vi "Wago 4 Station Door Status.vi"(7 "Station 1-4":bool, 8 "error in (no error)":errorcluster, 10 "Wago Data Input":T2 {"Input Process Image"."Software Constants"."Room PID Settings"."Room Dehumid Temperature I (*RM Dehum I1)" max=30000 step=1; "Input Process Image"."Software Constants"."Room PID Settings"."Room Dehumid Temperature P (*RM Dehum P1)" max=30000 step=1; "Input Process Image"."Software Constants"."Room PID Settings"."Room Cool Temperature I (*RM Cool I1)" max=30000 step=1; "Input Process Image"."Software Constants"."Room PID Settings"."Room Cool Temperature P (*RM Cool P1)" max=30000 step=1; "Input Process Image"."Software Constants"."Room PID Settings"."Room Heat I (*RM Heat I1)" max=30000 step=1; "Input Process Image"."Software Constants"."Room PID Settings"."Room Heat P (*RM Heat P1)" max=30000 step=1; "Input Process Image"."Software Constants"."Room PID Settings"."Room Humidity I (*RM Hum I1)" max=30000 step=1; "Input Process Image"."Software Constants"."Room PID Settings"."Room Humidity P (*RM Hum P1)" max=30000 step=1; "Input Process Image"."Software Constants"."Room PID Settings"."Room Dry I (*RM Dry I1)" max=30000 step=1; "Input Process Image"."Software Constants"."Room PID Settings"."Room Dry P(*RM Dry P1)" max=30000 step=1}, 11 "Modbus Master in":refnum<class "Modbus Master.lvclass">) -> (0 "error out":errorcluster, 2 "Wago Data Output":T2 {"Input Process Image"."Software Constants"."Room PID Settings"."Room Dehumid Temperature I (*RM Dehum I1)" max=30000 step=1; "Input Process Image"."Software Constants"."Room PID Settings"."Room Dehumid Temperature P (*RM Dehum P1)" max=30000 step=1; "Input Process Image"."Software Constants"."Room PID Settings"."Room Cool Temperature I (*RM Cool I1)" max=30000 step=1; "Input Process Image"."Software Constants"."Room PID Settings"."Room Cool Temperature P (*RM Cool P1)" max=30000 step=1; "Input Process Image"."Software Constants"."Room PID Settings"."Room Heat I (*RM Heat I1)" max=30000 step=1; "Input Process Image"."Software Constants"."Room PID Settings"."Room Heat P (*RM Heat P1)" max=30000 step=1; "Input Process Image"."Software Constants"."Room PID Settings"."Room Humidity I (*RM Hum I1)" max=30000 step=1; "Input Process Image"."Software Constants"."Room PID Settings"."Room Humidity P (*RM Hum P1)" max=30000 step=1; "Input Process Image"."Software Constants"."Room PID Settings"."Room Dry I (*RM Dry I1)" max=30000 step=1; "Input Process Image"."Software Constants"."Room PID Settings"."Room Dry P(*RM Dry P1)" max=30000 step=1}, 3 "Modbus master out":refnum<class "Modbus Master.lvclass">)   [LabVIEW 2016]
uses:
  <vilib>/NI/Modbus Library/API/Master/Modbus Master.lvclass
  Type Definitions/Wago Main Control.ctl
  Type Definitions/Wago Output Data Process Image.ctl
  Type Definitions/Wago Room Condtions.ctl
  Type Definitions/Wago Door Relays.ctl
  Type Definitions/Wago Contactor Settings.ctl
  Type Definitions/Wago Ground Leakage.ctl
  Type Definitions/Wago Input Process Image.ctl
  Type Definitions/Wago Room PID Settings.ctl
  Type Definitions/Wago Measured Input Data.ctl
  Type Definitions/Wago Room Setpoint Targets.ctl
  Type Definitions/Wago Output Commands.ctl
panel:
  in  "Wago Output Words 24":T1=839 items=["twHeatCtrl"=512, "twSteamCtrl"=513, "twCoolCtrl"=514, "twDehumCtrl"=515, "Output QX4 Bool"=516, "Output QX5 Bool"=517, "Output QX6 Bool"=518, "Output QX7 Bool"=519, "Output QX8 Bool"=520, "Output QX9 Bool"=521, "Output QX10"=522, "twRoomTemp"=840, "twRoomHum"=841, "twSuppTemp"=842, "twCoolTemp"=843, "twDehumTemp"=844, "twGlycolTemp"=845, "twHeatRate"=846, "twSteamRate"=847, "twCoolRate"=848, "twDehumRate"=849, "twStatus"=850, "twDoorEna"=851, "Rm1St1Dr1Stat"=816, "Rm1St2Dr1Stat"=817, "Rm1St3Dr1Stat"=818, "Rm1St4Dr1Stat"=819, "Rm1St5Dr1Stat"=820, "Rm1St6Dr1Stat"=821, "Rm1St7Dr1Stat"=822, "Rm1St8Dr1Stat"=823, "Rm1St1Dr2Stat"=824, "Rm1St2Dr2Stat"=825, "Rm1St3Dr2Stat"=826, "Rm1St4Dr2Stat"=827, "Rm1St5Dr2Stat"=828, "Rm1St6DrStat"=829, "Rm1St7Dr2Stat"=830, "Rm1St8Dr2Stat"=831, "Rm1St1Dr3Stat"=832, "Rm1St2Dr3Stat"=833, "Rm1St3Dr3Stat"=834, "Rm1St4Dr3Stat"=835, "Rm1St5Dr3Stat"=836, "Rm1St6Dr3Stat"=837, "Rm1St7Dr3Stat"=838, "Rm1St8Dr3Stat"=839, "twVoltMon1"=784, "twVoltMon2"=785, "twVoltMon3"=786, "twVoltMon4"=787, "twVoltMon5"=788, "twVoltMon6"=789, "twVoltMon7"=790, "twVoltMon8"=791, "twVoltStat1"=792, "twVoltStat2"=793, "twVoltStat3"=794, "twVoltStat4"=795, "twVoltStat5"=796, "twVoltStat6"=797, "twVoltStat7"=798, "twVoltStat8"=799]
  in  "Wago Output Words 23":T1=831 items=["twHeatCtrl"=512, "twSteamCtrl"=513, "twCoolCtrl"=514, "twDehumCtrl"=515, "Output QX4 Bool"=516, "Output QX5 Bool"=517, "Output QX6 Bool"=518, "Output QX7 Bool"=519, "Output QX8 Bool"=520, "Output QX9 Bool"=521, "Output QX10"=522, "twRoomTemp"=840, "twRoomHum"=841, "twSuppTemp"=842, "twCoolTemp"=843, "twDehumTemp"=844, "twGlycolTemp"=845, "twHeatRate"=846, "twSteamRate"=847, "twCoolRate"=848, "twDehumRate"=849, "twStatus"=850, "twDoorEna"=851, "Rm1St1Dr1Stat"=816, "Rm1St2Dr1Stat"=817, "Rm1St3Dr1Stat"=818, "Rm1St4Dr1Stat"=819, "Rm1St5Dr1Stat"=820, "Rm1St6Dr1Stat"=821, "Rm1St7Dr1Stat"=822, "Rm1St8Dr1Stat"=823, "Rm1St1Dr2Stat"=824, "Rm1St2Dr2Stat"=825, "Rm1St3Dr2Stat"=826, "Rm1St4Dr2Stat"=827, "Rm1St5Dr2Stat"=828, "Rm1St6DrStat"=829, "Rm1St7Dr2Stat"=830, "Rm1St8Dr2Stat"=831, "Rm1St1Dr3Stat"=832, "Rm1St2Dr3Stat"=833, "Rm1St3Dr3Stat"=834, "Rm1St4Dr3Stat"=835, "Rm1St5Dr3Stat"=836, "Rm1St6Dr3Stat"=837, "Rm1St7Dr3Stat"=838, "Rm1St8Dr3Stat"=839, "twVoltMon1"=784, "twVoltMon2"=785, "twVoltMon3"=786, "twVoltMon4"=787, "twVoltMon5"=788, "twVoltMon6"=789, "twVoltMon7"=790, "twVoltMon8"=791, "twVoltStat1"=792, "twVoltStat2"=793, "twVoltStat3"=794, "twVoltStat4"=795, "twVoltStat5"=796, "twVoltStat6"=797, "twVoltStat7"=798, "twVoltStat8"=799]
  in  "Wago Output Words 22":T1=823 items=["twHeatCtrl"=512, "twSteamCtrl"=513, "twCoolCtrl"=514, "twDehumCtrl"=515, "Output QX4 Bool"=516, "Output QX5 Bool"=517, "Output QX6 Bool"=518, "Output QX7 Bool"=519, "Output QX8 Bool"=520, "Output QX9 Bool"=521, "Output QX10"=522, "twRoomTemp"=840, "twRoomHum"=841, "twSuppTemp"=842, "twCoolTemp"=843, "twDehumTemp"=844, "twGlycolTemp"=845, "twHeatRate"=846, "twSteamRate"=847, "twCoolRate"=848, "twDehumRate"=849, "twStatus"=850, "twDoorEna"=851, "Rm1St1Dr1Stat"=816, "Rm1St2Dr1Stat"=817, "Rm1St3Dr1Stat"=818, "Rm1St4Dr1Stat"=819, "Rm1St5Dr1Stat"=820, "Rm1St6Dr1Stat"=821, "Rm1St7Dr1Stat"=822, "Rm1St8Dr1Stat"=823, "Rm1St1Dr2Stat"=824, "Rm1St2Dr2Stat"=825, "Rm1St3Dr2Stat"=826, "Rm1St4Dr2Stat"=827, "Rm1St5Dr2Stat"=828, "Rm1St6DrStat"=829, "Rm1St7Dr2Stat"=830, "Rm1St8Dr2Stat"=831, "Rm1St1Dr3Stat"=832, "Rm1St2Dr3Stat"=833, "Rm1St3Dr3Stat"=834, "Rm1St4Dr3Stat"=835, "Rm1St5Dr3Stat"=836, "Rm1St6Dr3Stat"=837, "Rm1St7Dr3Stat"=838, "Rm1St8Dr3Stat"=839, "twVoltMon1"=784, "twVoltMon2"=785, "twVoltMon3"=786, "twVoltMon4"=787, "twVoltMon5"=788, "twVoltMon6"=789, "twVoltMon7"=790, "twVoltMon8"=791, "twVoltStat1"=792, "twVoltStat2"=793, "twVoltStat3"=794, "twVoltStat4"=795, "twVoltStat5"=796, "twVoltStat6"=797, "twVoltStat7"=798, "twVoltStat8"=799]
  in  "Wago Output Words 21":T1=838 items=["twHeatCtrl"=512, "twSteamCtrl"=513, "twCoolCtrl"=514, "twDehumCtrl"=515, "Output QX4 Bool"=516, "Output QX5 Bool"=517, "Output QX6 Bool"=518, "Output QX7 Bool"=519, "Output QX8 Bool"=520, "Output QX9 Bool"=521, "Output QX10"=522, "twRoomTemp"=840, "twRoomHum"=841, "twSuppTemp"=842, "twCoolTemp"=843, "twDehumTemp"=844, "twGlycolTemp"=845, "twHeatRate"=846, "twSteamRate"=847, "twCoolRate"=848, "twDehumRate"=849, "twStatus"=850, "twDoorEna"=851, "Rm1St1Dr1Stat"=816, "Rm1St2Dr1Stat"=817, "Rm1St3Dr1Stat"=818, "Rm1St4Dr1Stat"=819, "Rm1St5Dr1Stat"=820, "Rm1St6Dr1Stat"=821, "Rm1St7Dr1Stat"=822, "Rm1St8Dr1Stat"=823, "Rm1St1Dr2Stat"=824, "Rm1St2Dr2Stat"=825, "Rm1St3Dr2Stat"=826, "Rm1St4Dr2Stat"=827, "Rm1St5Dr2Stat"=828, "Rm1St6DrStat"=829, "Rm1St7Dr2Stat"=830, "Rm1St8Dr2Stat"=831, "Rm1St1Dr3Stat"=832, "Rm1St2Dr3Stat"=833, "Rm1St3Dr3Stat"=834, "Rm1St4Dr3Stat"=835, "Rm1St5Dr3Stat"=836, "Rm1St6Dr3Stat"=837, "Rm1St7Dr3Stat"=838, "Rm1St8Dr3Stat"=839, "twVoltMon1"=784, "twVoltMon2"=785, "twVoltMon3"=786, "twVoltMon4"=787, "twVoltMon5"=788, "twVoltMon6"=789, "twVoltMon7"=790, "twVoltMon8"=791, "twVoltStat1"=792, "twVoltStat2"=793, "twVoltStat3"=794, "twVoltStat4"=795, "twVoltStat5"=796, "twVoltStat6"=797, "twVoltStat7"=798, "twVoltStat8"=799]
  in  "Wago Output Words 20":T1=830 items=["twHeatCtrl"=512, "twSteamCtrl"=513, "twCoolCtrl"=514, "twDehumCtrl"=515, "Output QX4 Bool"=516, "Output QX5 Bool"=517, "Output QX6 Bool"=518, "Output QX7 Bool"=519, "Output QX8 Bool"=520, "Output QX9 Bool"=521, "Output QX10"=522, "twRoomTemp"=840, "twRoomHum"=841, "twSuppTemp"=842, "twCoolTemp"=843, "twDehumTemp"=844, "twGlycolTemp"=845, "twHeatRate"=846, "twSteamRate"=847, "twCoolRate"=848, "twDehumRate"=849, "twStatus"=850, "twDoorEna"=851, "Rm1St1Dr1Stat"=816, "Rm1St2Dr1Stat"=817, "Rm1St3Dr1Stat"=818, "Rm1St4Dr1Stat"=819, "Rm1St5Dr1Stat"=820, "Rm1St6Dr1Stat"=821, "Rm1St7Dr1Stat"=822, "Rm1St8Dr1Stat"=823, "Rm1St1Dr2Stat"=824, "Rm1St2Dr2Stat"=825, "Rm1St3Dr2Stat"=826, "Rm1St4Dr2Stat"=827, "Rm1St5Dr2Stat"=828, "Rm1St6DrStat"=829, "Rm1St7Dr2Stat"=830, "Rm1St8Dr2Stat"=831, "Rm1St1Dr3Stat"=832, "Rm1St2Dr3Stat"=833, "Rm1St3Dr3Stat"=834, "Rm1St4Dr3Stat"=835, "Rm1St5Dr3Stat"=836, "Rm1St6Dr3Stat"=837, "Rm1St7Dr3Stat"=838, "Rm1St8Dr3Stat"=839, "twVoltMon1"=784, "twVoltMon2"=785, "twVoltMon3"=786, "twVoltMon4"=787, "twVoltMon5"=788, "twVoltMon6"=789, "twVoltMon7"=790, "twVoltMon8"=791, "twVoltStat1"=792, "twVoltStat2"=793, "twVoltStat3"=794, "twVoltStat4"=795, "twVoltStat5"=796, "twVoltStat6"=797, "twVoltStat7"=798, "twVoltStat8"=799]
  in  "Wago Output Words 19":T1=822 items=["twHeatCtrl"=512, "twSteamCtrl"=513, "twCoolCtrl"=514, "twDehumCtrl"=515, "Output QX4 Bool"=516, "Output QX5 Bool"=517, "Output QX6 Bool"=518, "Output QX7 Bool"=519, "Output QX8 Bool"=520, "Output QX9 Bool"=521, "Output QX10"=522, "twRoomTemp"=840, "twRoomHum"=841, "twSuppTemp"=842, "twCoolTemp"=843, "twDehumTemp"=844, "twGlycolTemp"=845, "twHeatRate"=846, "twSteamRate"=847, "twCoolRate"=848, "twDehumRate"=849, "twStatus"=850, "twDoorEna"=851, "Rm1St1Dr1Stat"=816, "Rm1St2Dr1Stat"=817, "Rm1St3Dr1Stat"=818, "Rm1St4Dr1Stat"=819, "Rm1St5Dr1Stat"=820, "Rm1St6Dr1Stat"=821, "Rm1St7Dr1Stat"=822, "Rm1St8Dr1Stat"=823, "Rm1St1Dr2Stat"=824, "Rm1St2Dr2Stat"=825, "Rm1St3Dr2Stat"=826, "Rm1St4Dr2Stat"=827, "Rm1St5Dr2Stat"=828, "Rm1St6DrStat"=829, "Rm1St7Dr2Stat"=830, "Rm1St8Dr2Stat"=831, "Rm1St1Dr3Stat"=832, "Rm1St2Dr3Stat"=833, "Rm1St3Dr3Stat"=834, "Rm1St4Dr3Stat"=835, "Rm1St5Dr3Stat"=836, "Rm1St6Dr3Stat"=837, "Rm1St7Dr3Stat"=838, "Rm1St8Dr3Stat"=839, "twVoltMon1"=784, "twVoltMon2"=785, "twVoltMon3"=786, "twVoltMon4"=787, "twVoltMon5"=788, "twVoltMon6"=789, "twVoltMon7"=790, "twVoltMon8"=791, "twVoltStat1"=792, "twVoltStat2"=793, "twVoltStat3"=794, "twVoltStat4"=795, "twVoltStat5"=796, "twVoltStat6"=797, "twVoltStat7"=798, "twVoltStat8"=799]
  in  "Wago Output Words 18":T1=837 items=["twHeatCtrl"=512, "twSteamCtrl"=513, "twCoolCtrl"=514, "twDehumCtrl"=515, "Output QX4 Bool"=516, "Output QX5 Bool"=517, "Output QX6 Bool"=518, "Output QX7 Bool"=519, "Output QX8 Bool"=520, "Output QX9 Bool"=521, "Output QX10"=522, "twRoomTemp"=840, "twRoomHum"=841, "twSuppTemp"=842, "twCoolTemp"=843, "twDehumTemp"=844, "twGlycolTemp"=845, "twHeatRate"=846, "twSteamRate"=847, "twCoolRate"=848, "twDehumRate"=849, "twStatus"=850, "twDoorEna"=851, "Rm1St1Dr1Stat"=816, "Rm1St2Dr1Stat"=817, "Rm1St3Dr1Stat"=818, "Rm1St4Dr1Stat"=819, "Rm1St5Dr1Stat"=820, "Rm1St6Dr1Stat"=821, "Rm1St7Dr1Stat"=822, "Rm1St8Dr1Stat"=823, "Rm1St1Dr2Stat"=824, "Rm1St2Dr2Stat"=825, "Rm1St3Dr2Stat"=826, "Rm1St4Dr2Stat"=827, "Rm1St5Dr2Stat"=828, "Rm1St6DrStat"=829, "Rm1St7Dr2Stat"=830, "Rm1St8Dr2Stat"=831, "Rm1St1Dr3Stat"=832, "Rm1St2Dr3Stat"=833, "Rm1St3Dr3Stat"=834, "Rm1St4Dr3Stat"=835, "Rm1St5Dr3Stat"=836, "Rm1St6Dr3Stat"=837, "Rm1St7Dr3Stat"=838, "Rm1St8Dr3Stat"=839, "twVoltMon1"=784, "twVoltMon2"=785, "twVoltMon3"=786, "twVoltMon4"=787, "twVoltMon5"=788, "twVoltMon6"=789, "twVoltMon7"=790, "twVoltMon8"=791, "twVoltStat1"=792, "twVoltStat2"=793, "twVoltStat3"=794, "twVoltStat4"=795, "twVoltStat5"=796, "twVoltStat6"=797, "twVoltStat7"=798, "twVoltStat8"=799]
  in  "Wago Output Words 17":T1=829 items=["twHeatCtrl"=512, "twSteamCtrl"=513, "twCoolCtrl"=514, "twDehumCtrl"=515, "Output QX4 Bool"=516, "Output QX5 Bool"=517, "Output QX6 Bool"=518, "Output QX7 Bool"=519, "Output QX8 Bool"=520, "Output QX9 Bool"=521, "Output QX10"=522, "twRoomTemp"=840, "twRoomHum"=841, "twSuppTemp"=842, "twCoolTemp"=843, "twDehumTemp"=844, "twGlycolTemp"=845, "twHeatRate"=846, "twSteamRate"=847, "twCoolRate"=848, "twDehumRate"=849, "twStatus"=850, "twDoorEna"=851, "Rm1St1Dr1Stat"=816, "Rm1St2Dr1Stat"=817, "Rm1St3Dr1Stat"=818, "Rm1St4Dr1Stat"=819, "Rm1St5Dr1Stat"=820, "Rm1St6Dr1Stat"=821, "Rm1St7Dr1Stat"=822, "Rm1St8Dr1Stat"=823, "Rm1St1Dr2Stat"=824, "Rm1St2Dr2Stat"=825, "Rm1St3Dr2Stat"=826, "Rm1St4Dr2Stat"=827, "Rm1St5Dr2Stat"=828, "Rm1St6DrStat"=829, "Rm1St7Dr2Stat"=830, "Rm1St8Dr2Stat"=831, "Rm1St1Dr3Stat"=832, "Rm1St2Dr3Stat"=833, "Rm1St3Dr3Stat"=834, "Rm1St4Dr3Stat"=835, "Rm1St5Dr3Stat"=836, "Rm1St6Dr3Stat"=837, "Rm1St7Dr3Stat"=838, "Rm1St8Dr3Stat"=839, "twVoltMon1"=784, "twVoltMon2"=785, "twVoltMon3"=786, "twVoltMon4"=787, "twVoltMon5"=788, "twVoltMon6"=789, "twVoltMon7"=790, "twVoltMon8"=791, "twVoltStat1"=792, "twVoltStat2"=793, "twVoltStat3"=794, "twVoltStat4"=795, "twVoltStat5"=796, "twVoltStat6"=797, "twVoltStat7"=798, "twVoltStat8"=799]
  in  "Wago Output Words 16":T1=821 items=["twHeatCtrl"=512, "twSteamCtrl"=513, "twCoolCtrl"=514, "twDehumCtrl"=515, "Output QX4 Bool"=516, "Output QX5 Bool"=517, "Output QX6 Bool"=518, "Output QX7 Bool"=519, "Output QX8 Bool"=520, "Output QX9 Bool"=521, "Output QX10"=522, "twRoomTemp"=840, "twRoomHum"=841, "twSuppTemp"=842, "twCoolTemp"=843, "twDehumTemp"=844, "twGlycolTemp"=845, "twHeatRate"=846, "twSteamRate"=847, "twCoolRate"=848, "twDehumRate"=849, "twStatus"=850, "twDoorEna"=851, "Rm1St1Dr1Stat"=816, "Rm1St2Dr1Stat"=817, "Rm1St3Dr1Stat"=818, "Rm1St4Dr1Stat"=819, "Rm1St5Dr1Stat"=820, "Rm1St6Dr1Stat"=821, "Rm1St7Dr1Stat"=822, "Rm1St8Dr1Stat"=823, "Rm1St1Dr2Stat"=824, "Rm1St2Dr2Stat"=825, "Rm1St3Dr2Stat"=826, "Rm1St4Dr2Stat"=827, "Rm1St5Dr2Stat"=828, "Rm1St6DrStat"=829, "Rm1St7Dr2Stat"=830, "Rm1St8Dr2Stat"=831, "Rm1St1Dr3Stat"=832, "Rm1St2Dr3Stat"=833, "Rm1St3Dr3Stat"=834, "Rm1St4Dr3Stat"=835, "Rm1St5Dr3Stat"=836, "Rm1St6Dr3Stat"=837, "Rm1St7Dr3Stat"=838, "Rm1St8Dr3Stat"=839, "twVoltMon1"=784, "twVoltMon2"=785, "twVoltMon3"=786, "twVoltMon4"=787, "twVoltMon5"=788, "twVoltMon6"=789, "twVoltMon7"=790, "twVoltMon8"=791, "twVoltStat1"=792, "twVoltStat2"=793, "twVoltStat3"=794, "twVoltStat4"=795, "twVoltStat5"=796, "twVoltStat6"=797, "twVoltStat7"=798, "twVoltStat8"=799]
  in  "Wago Output Words 15":T1=836 items=["twHeatCtrl"=512, "twSteamCtrl"=513, "twCoolCtrl"=514, "twDehumCtrl"=515, "Output QX4 Bool"=516, "Output QX5 Bool"=517, "Output QX6 Bool"=518, "Output QX7 Bool"=519, "Output QX8 Bool"=520, "Output QX9 Bool"=521, "Output QX10"=522, "twRoomTemp"=840, "twRoomHum"=841, "twSuppTemp"=842, "twCoolTemp"=843, "twDehumTemp"=844, "twGlycolTemp"=845, "twHeatRate"=846, "twSteamRate"=847, "twCoolRate"=848, "twDehumRate"=849, "twStatus"=850, "twDoorEna"=851, "Rm1St1Dr1Stat"=816, "Rm1St2Dr1Stat"=817, "Rm1St3Dr1Stat"=818, "Rm1St4Dr1Stat"=819, "Rm1St5Dr1Stat"=820, "Rm1St6Dr1Stat"=821, "Rm1St7Dr1Stat"=822, "Rm1St8Dr1Stat"=823, "Rm1St1Dr2Stat"=824, "Rm1St2Dr2Stat"=825, "Rm1St3Dr2Stat"=826, "Rm1St4Dr2Stat"=827, "Rm1St5Dr2Stat"=828, "Rm1St6DrStat"=829, "Rm1St7Dr2Stat"=830, "Rm1St8Dr2Stat"=831, "Rm1St1Dr3Stat"=832, "Rm1St2Dr3Stat"=833, "Rm1St3Dr3Stat"=834, "Rm1St4Dr3Stat"=835, "Rm1St5Dr3Stat"=836, "Rm1St6Dr3Stat"=837, "Rm1St7Dr3Stat"=838, "Rm1St8Dr3Stat"=839, "twVoltMon1"=784, "twVoltMon2"=785, "twVoltMon3"=786, "twVoltMon4"=787, "twVoltMon5"=788, "twVoltMon6"=789, "twVoltMon7"=790, "twVoltMon8"=791, "twVoltStat1"=792, "twVoltStat2"=793, "twVoltStat3"=794, "twVoltStat4"=795, "twVoltStat5"=796, "twVoltStat6"=797, "twVoltStat7"=798, "twVoltStat8"=799]
  in  "Wago Output Words 14":T1=828 items=["twHeatCtrl"=512, "twSteamCtrl"=513, "twCoolCtrl"=514, "twDehumCtrl"=515, "Output QX4 Bool"=516, "Output QX5 Bool"=517, "Output QX6 Bool"=518, "Output QX7 Bool"=519, "Output QX8 Bool"=520, "Output QX9 Bool"=521, "Output QX10"=522, "twRoomTemp"=840, "twRoomHum"=841, "twSuppTemp"=842, "twCoolTemp"=843, "twDehumTemp"=844, "twGlycolTemp"=845, "twHeatRate"=846, "twSteamRate"=847, "twCoolRate"=848, "twDehumRate"=849, "twStatus"=850, "twDoorEna"=851, "Rm1St1Dr1Stat"=816, "Rm1St2Dr1Stat"=817, "Rm1St3Dr1Stat"=818, "Rm1St4Dr1Stat"=819, "Rm1St5Dr1Stat"=820, "Rm1St6Dr1Stat"=821, "Rm1St7Dr1Stat"=822, "Rm1St8Dr1Stat"=823, "Rm1St1Dr2Stat"=824, "Rm1St2Dr2Stat"=825, "Rm1St3Dr2Stat"=826, "Rm1St4Dr2Stat"=827, "Rm1St5Dr2Stat"=828, "Rm1St6DrStat"=829, "Rm1St7Dr2Stat"=830, "Rm1St8Dr2Stat"=831, "Rm1St1Dr3Stat"=832, "Rm1St2Dr3Stat"=833, "Rm1St3Dr3Stat"=834, "Rm1St4Dr3Stat"=835, "Rm1St5Dr3Stat"=836, "Rm1St6Dr3Stat"=837, "Rm1St7Dr3Stat"=838, "Rm1St8Dr3Stat"=839, "twVoltMon1"=784, "twVoltMon2"=785, "twVoltMon3"=786, "twVoltMon4"=787, "twVoltMon5"=788, "twVoltMon6"=789, "twVoltMon7"=790, "twVoltMon8"=791, "twVoltStat1"=792, "twVoltStat2"=793, "twVoltStat3"=794, "twVoltStat4"=795, "twVoltStat5"=796, "twVoltStat6"=797, "twVoltStat7"=798, "twVoltStat8"=799]
  in  "Wago Output Words 13":T1=820 items=["twHeatCtrl"=512, "twSteamCtrl"=513, "twCoolCtrl"=514, "twDehumCtrl"=515, "Output QX4 Bool"=516, "Output QX5 Bool"=517, "Output QX6 Bool"=518, "Output QX7 Bool"=519, "Output QX8 Bool"=520, "Output QX9 Bool"=521, "Output QX10"=522, "twRoomTemp"=840, "twRoomHum"=841, "twSuppTemp"=842, "twCoolTemp"=843, "twDehumTemp"=844, "twGlycolTemp"=845, "twHeatRate"=846, "twSteamRate"=847, "twCoolRate"=848, "twDehumRate"=849, "twStatus"=850, "twDoorEna"=851, "Rm1St1Dr1Stat"=816, "Rm1St2Dr1Stat"=817, "Rm1St3Dr1Stat"=818, "Rm1St4Dr1Stat"=819, "Rm1St5Dr1Stat"=820, "Rm1St6Dr1Stat"=821, "Rm1St7Dr1Stat"=822, "Rm1St8Dr1Stat"=823, "Rm1St1Dr2Stat"=824, "Rm1St2Dr2Stat"=825, "Rm1St3Dr2Stat"=826, "Rm1St4Dr2Stat"=827, "Rm1St5Dr2Stat"=828, "Rm1St6DrStat"=829, "Rm1St7Dr2Stat"=830, "Rm1St8Dr2Stat"=831, "Rm1St1Dr3Stat"=832, "Rm1St2Dr3Stat"=833, "Rm1St3Dr3Stat"=834, "Rm1St4Dr3Stat"=835, "Rm1St5Dr3Stat"=836, "Rm1St6Dr3Stat"=837, "Rm1St7Dr3Stat"=838, "Rm1St8Dr3Stat"=839, "twVoltMon1"=784, "twVoltMon2"=785, "twVoltMon3"=786, "twVoltMon4"=787, "twVoltMon5"=788, "twVoltMon6"=789, "twVoltMon7"=790, "twVoltMon8"=791, "twVoltStat1"=792, "twVoltStat2"=793, "twVoltStat3"=794, "twVoltStat4"=795, "twVoltStat5"=796, "twVoltStat6"=797, "twVoltStat7"=798, "twVoltStat8"=799]
  in  "Wago Output Words 12":T1=835 items=["twHeatCtrl"=512, "twSteamCtrl"=513, "twCoolCtrl"=514, "twDehumCtrl"=515, "Output QX4 Bool"=516, "Output QX5 Bool"=517, "Output QX6 Bool"=518, "Output QX7 Bool"=519, "Output QX8 Bool"=520, "Output QX9 Bool"=521, "Output QX10"=522, "twRoomTemp"=840, "twRoomHum"=841, "twSuppTemp"=842, "twCoolTemp"=843, "twDehumTemp"=844, "twGlycolTemp"=845, "twHeatRate"=846, "twSteamRate"=847, "twCoolRate"=848, "twDehumRate"=849, "twStatus"=850, "twDoorEna"=851, "Rm1St1Dr1Stat"=816, "Rm1St2Dr1Stat"=817, "Rm1St3Dr1Stat"=818, "Rm1St4Dr1Stat"=819, "Rm1St5Dr1Stat"=820, "Rm1St6Dr1Stat"=821, "Rm1St7Dr1Stat"=822, "Rm1St8Dr1Stat"=823, "Rm1St1Dr2Stat"=824, "Rm1St2Dr2Stat"=825, "Rm1St3Dr2Stat"=826, "Rm1St4Dr2Stat"=827, "Rm1St5Dr2Stat"=828, "Rm1St6DrStat"=829, "Rm1St7Dr2Stat"=830, "Rm1St8Dr2Stat"=831, "Rm1St1Dr3Stat"=832, "Rm1St2Dr3Stat"=833, "Rm1St3Dr3Stat"=834, "Rm1St4Dr3Stat"=835, "Rm1St5Dr3Stat"=836, "Rm1St6Dr3Stat"=837, "Rm1St7Dr3Stat"=838, "Rm1St8Dr3Stat"=839, "twVoltMon1"=784, "twVoltMon2"=785, "twVoltMon3"=786, "twVoltMon4"=787, "twVoltMon5"=788, "twVoltMon6"=789, "twVoltMon7"=790, "twVoltMon8"=791, "twVoltStat1"=792, "twVoltStat2"=793, "twVoltStat3"=794, "twVoltStat4"=795, "twVoltStat5"=796, "twVoltStat6"=797, "twVoltStat7"=798, "twVoltStat8"=799]
  in  "Wago Output Words 11":T1=827 items=["twHeatCtrl"=512, "twSteamCtrl"=513, "twCoolCtrl"=514, "twDehumCtrl"=515, "Output QX4 Bool"=516, "Output QX5 Bool"=517, "Output QX6 Bool"=518, "Output QX7 Bool"=519, "Output QX8 Bool"=520, "Output QX9 Bool"=521, "Output QX10"=522, "twRoomTemp"=840, "twRoomHum"=841, "twSuppTemp"=842, "twCoolTemp"=843, "twDehumTemp"=844, "twGlycolTemp"=845, "twHeatRate"=846, "twSteamRate"=847, "twCoolRate"=848, "twDehumRate"=849, "twStatus"=850, "twDoorEna"=851, "Rm1St1Dr1Stat"=816, "Rm1St2Dr1Stat"=817, "Rm1St3Dr1Stat"=818, "Rm1St4Dr1Stat"=819, "Rm1St5Dr1Stat"=820, "Rm1St6Dr1Stat"=821, "Rm1St7Dr1Stat"=822, "Rm1St8Dr1Stat"=823, "Rm1St1Dr2Stat"=824, "Rm1St2Dr2Stat"=825, "Rm1St3Dr2Stat"=826, "Rm1St4Dr2Stat"=827, "Rm1St5Dr2Stat"=828, "Rm1St6DrStat"=829, "Rm1St7Dr2Stat"=830, "Rm1St8Dr2Stat"=831, "Rm1St1Dr3Stat"=832, "Rm1St2Dr3Stat"=833, "Rm1St3Dr3Stat"=834, "Rm1St4Dr3Stat"=835, "Rm1St5Dr3Stat"=836, "Rm1St6Dr3Stat"=837, "Rm1St7Dr3Stat"=838, "Rm1St8Dr3Stat"=839, "twVoltMon1"=784, "twVoltMon2"=785, "twVoltMon3"=786, "twVoltMon4"=787, "twVoltMon5"=788, "twVoltMon6"=789, "twVoltMon7"=790, "twVoltMon8"=791, "twVoltStat1"=792, "twVoltStat2"=793, "twVoltStat3"=794, "twVoltStat4"=795, "twVoltStat5"=796, "twVoltStat6"=797, "twVoltStat7"=798, "twVoltStat8"=799]
  in  "Wago Output Words 10":T1=819 items=["twHeatCtrl"=512, "twSteamCtrl"=513, "twCoolCtrl"=514, "twDehumCtrl"=515, "Output QX4 Bool"=516, "Output QX5 Bool"=517, "Output QX6 Bool"=518, "Output QX7 Bool"=519, "Output QX8 Bool"=520, "Output QX9 Bool"=521, "Output QX10"=522, "twRoomTemp"=840, "twRoomHum"=841, "twSuppTemp"=842, "twCoolTemp"=843, "twDehumTemp"=844, "twGlycolTemp"=845, "twHeatRate"=846, "twSteamRate"=847, "twCoolRate"=848, "twDehumRate"=849, "twStatus"=850, "twDoorEna"=851, "Rm1St1Dr1Stat"=816, "Rm1St2Dr1Stat"=817, "Rm1St3Dr1Stat"=818, "Rm1St4Dr1Stat"=819, "Rm1St5Dr1Stat"=820, "Rm1St6Dr1Stat"=821, "Rm1St7Dr1Stat"=822, "Rm1St8Dr1Stat"=823, "Rm1St1Dr2Stat"=824, "Rm1St2Dr2Stat"=825, "Rm1St3Dr2Stat"=826, "Rm1St4Dr2Stat"=827, "Rm1St5Dr2Stat"=828, "Rm1St6DrStat"=829, "Rm1St7Dr2Stat"=830, "Rm1St8Dr2Stat"=831, "Rm1St1Dr3Stat"=832, "Rm1St2Dr3Stat"=833, "Rm1St3Dr3Stat"=834, "Rm1St4Dr3Stat"=835, "Rm1St5Dr3Stat"=836, "Rm1St6Dr3Stat"=837, "Rm1St7Dr3Stat"=838, "Rm1St8Dr3Stat"=839, "twVoltMon1"=784, "twVoltMon2"=785, "twVoltMon3"=786, "twVoltMon4"=787, "twVoltMon5"=788, "twVoltMon6"=789, "twVoltMon7"=790, "twVoltMon8"=791, "twVoltStat1"=792, "twVoltStat2"=793, "twVoltStat3"=794, "twVoltStat4"=795, "twVoltStat5"=796, "twVoltStat6"=797, "twVoltStat7"=798, "twVoltStat8"=799]
  in  "Wago Output Words 9":T1=834 items=["twHeatCtrl"=512, "twSteamCtrl"=513, "twCoolCtrl"=514, "twDehumCtrl"=515, "Output QX4 Bool"=516, "Output QX5 Bool"=517, "Output QX6 Bool"=518, "Output QX7 Bool"=519, "Output QX8 Bool"=520, "Output QX9 Bool"=521, "Output QX10"=522, "twRoomTemp"=840, "twRoomHum"=841, "twSuppTemp"=842, "twCoolTemp"=843, "twDehumTemp"=844, "twGlycolTemp"=845, "twHeatRate"=846, "twSteamRate"=847, "twCoolRate"=848, "twDehumRate"=849, "twStatus"=850, "twDoorEna"=851, "Rm1St1Dr1Stat"=816, "Rm1St2Dr1Stat"=817, "Rm1St3Dr1Stat"=818, "Rm1St4Dr1Stat"=819, "Rm1St5Dr1Stat"=820, "Rm1St6Dr1Stat"=821, "Rm1St7Dr1Stat"=822, "Rm1St8Dr1Stat"=823, "Rm1St1Dr2Stat"=824, "Rm1St2Dr2Stat"=825, "Rm1St3Dr2Stat"=826, "Rm1St4Dr2Stat"=827, "Rm1St5Dr2Stat"=828, "Rm1St6DrStat"=829, "Rm1St7Dr2Stat"=830, "Rm1St8Dr2Stat"=831, "Rm1St1Dr3Stat"=832, "Rm1St2Dr3Stat"=833, "Rm1St3Dr3Stat"=834, "Rm1St4Dr3Stat"=835, "Rm1St5Dr3Stat"=836, "Rm1St6Dr3Stat"=837, "Rm1St7Dr3Stat"=838, "Rm1St8Dr3Stat"=839, "twVoltMon1"=784, "twVoltMon2"=785, "twVoltMon3"=786, "twVoltMon4"=787, "twVoltMon5"=788, "twVoltMon6"=789, "twVoltMon7"=790, "twVoltMon8"=791, "twVoltStat1"=792, "twVoltStat2"=793, "twVoltStat3"=794, "twVoltStat4"=795, "twVoltStat5"=796, "twVoltStat6"=797, "twVoltStat7"=798, "twVoltStat8"=799]
  in  "Wago Output Words 8":T1=826 items=["twHeatCtrl"=512, "twSteamCtrl"=513, "twCoolCtrl"=514, "twDehumCtrl"=515, "Output QX4 Bool"=516, "Output QX5 Bool"=517, "Output QX6 Bool"=518, "Output QX7 Bool"=519, "Output QX8 Bool"=520, "Output QX9 Bool"=521, "Output QX10"=522, "twRoomTemp"=840, "twRoomHum"=841, "twSuppTemp"=842, "twCoolTemp"=843, "twDehumTemp"=844, "twGlycolTemp"=845, "twHeatRate"=846, "twSteamRate"=847, "twCoolRate"=848, "twDehumRate"=849, "twStatus"=850, "twDoorEna"=851, "Rm1St1Dr1Stat"=816, "Rm1St2Dr1Stat"=817, "Rm1St3Dr1Stat"=818, "Rm1St4Dr1Stat"=819, "Rm1St5Dr1Stat"=820, "Rm1St6Dr1Stat"=821, "Rm1St7Dr1Stat"=822, "Rm1St8Dr1Stat"=823, "Rm1St1Dr2Stat"=824, "Rm1St2Dr2Stat"=825, "Rm1St3Dr2Stat"=826, "Rm1St4Dr2Stat"=827, "Rm1St5Dr2Stat"=828, "Rm1St6DrStat"=829, "Rm1St7Dr2Stat"=830, "Rm1St8Dr2Stat"=831, "Rm1St1Dr3Stat"=832, "Rm1St2Dr3Stat"=833, "Rm1St3Dr3Stat"=834, "Rm1St4Dr3Stat"=835, "Rm1St5Dr3Stat"=836, "Rm1St6Dr3Stat"=837, "Rm1St7Dr3Stat"=838, "Rm1St8Dr3Stat"=839, "twVoltMon1"=784, "twVoltMon2"=785, "twVoltMon3"=786, "twVoltMon4"=787, "twVoltMon5"=788, "twVoltMon6"=789, "twVoltMon7"=790, "twVoltMon8"=791, "twVoltStat1"=792, "twVoltStat2"=793, "twVoltStat3"=794, "twVoltStat4"=795, "twVoltStat5"=796, "twVoltStat6"=797, "twVoltStat7"=798, "twVoltStat8"=799]
  in  "Wago Output Words 7":T1=818 items=["twHeatCtrl"=512, "twSteamCtrl"=513, "twCoolCtrl"=514, "twDehumCtrl"=515, "Output QX4 Bool"=516, "Output QX5 Bool"=517, "Output QX6 Bool"=518, "Output QX7 Bool"=519, "Output QX8 Bool"=520, "Output QX9 Bool"=521, "Output QX10"=522, "twRoomTemp"=840, "twRoomHum"=841, "twSuppTemp"=842, "twCoolTemp"=843, "twDehumTemp"=844, "twGlycolTemp"=845, "twHeatRate"=846, "twSteamRate"=847, "twCoolRate"=848, "twDehumRate"=849, "twStatus"=850, "twDoorEna"=851, "Rm1St1Dr1Stat"=816, "Rm1St2Dr1Stat"=817, "Rm1St3Dr1Stat"=818, "Rm1St4Dr1Stat"=819, "Rm1St5Dr1Stat"=820, "Rm1St6Dr1Stat"=821, "Rm1St7Dr1Stat"=822, "Rm1St8Dr1Stat"=823, "Rm1St1Dr2Stat"=824, "Rm1St2Dr2Stat"=825, "Rm1St3Dr2Stat"=826, "Rm1St4Dr2Stat"=827, "Rm1St5Dr2Stat"=828, "Rm1St6DrStat"=829, "Rm1St7Dr2Stat"=830, "Rm1St8Dr2Stat"=831, "Rm1St1Dr3Stat"=832, "Rm1St2Dr3Stat"=833, "Rm1St3Dr3Stat"=834, "Rm1St4Dr3Stat"=835, "Rm1St5Dr3Stat"=836, "Rm1St6Dr3Stat"=837, "Rm1St7Dr3Stat"=838, "Rm1St8Dr3Stat"=839, "twVoltMon1"=784, "twVoltMon2"=785, "twVoltMon3"=786, "twVoltMon4"=787, "twVoltMon5"=788, "twVoltMon6"=789, "twVoltMon7"=790, "twVoltMon8"=791, "twVoltStat1"=792, "twVoltStat2"=793, "twVoltStat3"=794, "twVoltStat4"=795, "twVoltStat5"=796, "twVoltStat6"=797, "twVoltStat7"=798, "twVoltStat8"=799]
  in  "Wago Output Words 6":T1=833 items=["twHeatCtrl"=512, "twSteamCtrl"=513, "twCoolCtrl"=514, "twDehumCtrl"=515, "Output QX4 Bool"=516, "Output QX5 Bool"=517, "Output QX6 Bool"=518, "Output QX7 Bool"=519, "Output QX8 Bool"=520, "Output QX9 Bool"=521, "Output QX10"=522, "twRoomTemp"=840, "twRoomHum"=841, "twSuppTemp"=842, "twCoolTemp"=843, "twDehumTemp"=844, "twGlycolTemp"=845, "twHeatRate"=846, "twSteamRate"=847, "twCoolRate"=848, "twDehumRate"=849, "twStatus"=850, "twDoorEna"=851, "Rm1St1Dr1Stat"=816, "Rm1St2Dr1Stat"=817, "Rm1St3Dr1Stat"=818, "Rm1St4Dr1Stat"=819, "Rm1St5Dr1Stat"=820, "Rm1St6Dr1Stat"=821, "Rm1St7Dr1Stat"=822, "Rm1St8Dr1Stat"=823, "Rm1St1Dr2Stat"=824, "Rm1St2Dr2Stat"=825, "Rm1St3Dr2Stat"=826, "Rm1St4Dr2Stat"=827, "Rm1St5Dr2Stat"=828, "Rm1St6DrStat"=829, "Rm1St7Dr2Stat"=830, "Rm1St8Dr2Stat"=831, "Rm1St1Dr3Stat"=832, "Rm1St2Dr3Stat"=833, "Rm1St3Dr3Stat"=834, "Rm1St4Dr3Stat"=835, "Rm1St5Dr3Stat"=836, "Rm1St6Dr3Stat"=837, "Rm1St7Dr3Stat"=838, "Rm1St8Dr3Stat"=839, "twVoltMon1"=784, "twVoltMon2"=785, "twVoltMon3"=786, "twVoltMon4"=787, "twVoltMon5"=788, "twVoltMon6"=789, "twVoltMon7"=790, "twVoltMon8"=791, "twVoltStat1"=792, "twVoltStat2"=793, "twVoltStat3"=794, "twVoltStat4"=795, "twVoltStat5"=796, "twVoltStat6"=797, "twVoltStat7"=798, "twVoltStat8"=799]
  in  "Wago Output Words 5":T1=825 items=["twHeatCtrl"=512, "twSteamCtrl"=513, "twCoolCtrl"=514, "twDehumCtrl"=515, "Output QX4 Bool"=516, "Output QX5 Bool"=517, "Output QX6 Bool"=518, "Output QX7 Bool"=519, "Output QX8 Bool"=520, "Output QX9 Bool"=521, "Output QX10"=522, "twRoomTemp"=840, "twRoomHum"=841, "twSuppTemp"=842, "twCoolTemp"=843, "twDehumTemp"=844, "twGlycolTemp"=845, "twHeatRate"=846, "twSteamRate"=847, "twCoolRate"=848, "twDehumRate"=849, "twStatus"=850, "twDoorEna"=851, "Rm1St1Dr1Stat"=816, "Rm1St2Dr1Stat"=817, "Rm1St3Dr1Stat"=818, "Rm1St4Dr1Stat"=819, "Rm1St5Dr1Stat"=820, "Rm1St6Dr1Stat"=821, "Rm1St7Dr1Stat"=822, "Rm1St8Dr1Stat"=823, "Rm1St1Dr2Stat"=824, "Rm1St2Dr2Stat"=825, "Rm1St3Dr2Stat"=826, "Rm1St4Dr2Stat"=827, "Rm1St5Dr2Stat"=828, "Rm1St6DrStat"=829, "Rm1St7Dr2Stat"=830, "Rm1St8Dr2Stat"=831, "Rm1St1Dr3Stat"=832, "Rm1St2Dr3Stat"=833, "Rm1St3Dr3Stat"=834, "Rm1St4Dr3Stat"=835, "Rm1St5Dr3Stat"=836, "Rm1St6Dr3Stat"=837, "Rm1St7Dr3Stat"=838, "Rm1St8Dr3Stat"=839, "twVoltMon1"=784, "twVoltMon2"=785, "twVoltMon3"=786, "twVoltMon4"=787, "twVoltMon5"=788, "twVoltMon6"=789, "twVoltMon7"=790, "twVoltMon8"=791, "twVoltStat1"=792, "twVoltStat2"=793, "twVoltStat3"=794, "twVoltStat4"=795, "twVoltStat5"=796, "twVoltStat6"=797, "twVoltStat7"=798, "twVoltStat8"=799]
  in  "Wago Output Words 4":T1=817 items=["twHeatCtrl"=512, "twSteamCtrl"=513, "twCoolCtrl"=514, "twDehumCtrl"=515, "Output QX4 Bool"=516, "Output QX5 Bool"=517, "Output QX6 Bool"=518, "Output QX7 Bool"=519, "Output QX8 Bool"=520, "Output QX9 Bool"=521, "Output QX10"=522, "twRoomTemp"=840, "twRoomHum"=841, "twSuppTemp"=842, "twCoolTemp"=843, "twDehumTemp"=844, "twGlycolTemp"=845, "twHeatRate"=846, "twSteamRate"=847, "twCoolRate"=848, "twDehumRate"=849, "twStatus"=850, "twDoorEna"=851, "Rm1St1Dr1Stat"=816, "Rm1St2Dr1Stat"=817, "Rm1St3Dr1Stat"=818, "Rm1St4Dr1Stat"=819, "Rm1St5Dr1Stat"=820, "Rm1St6Dr1Stat"=821, "Rm1St7Dr1Stat"=822, "Rm1St8Dr1Stat"=823, "Rm1St1Dr2Stat"=824, "Rm1St2Dr2Stat"=825, "Rm1St3Dr2Stat"=826, "Rm1St4Dr2Stat"=827, "Rm1St5Dr2Stat"=828, "Rm1St6DrStat"=829, "Rm1St7Dr2Stat"=830, "Rm1St8Dr2Stat"=831, "Rm1St1Dr3Stat"=832, "Rm1St2Dr3Stat"=833, "Rm1St3Dr3Stat"=834, "Rm1St4Dr3Stat"=835, "Rm1St5Dr3Stat"=836, "Rm1St6Dr3Stat"=837, "Rm1St7Dr3Stat"=838, "Rm1St8Dr3Stat"=839, "twVoltMon1"=784, "twVoltMon2"=785, "twVoltMon3"=786, "twVoltMon4"=787, "twVoltMon5"=788, "twVoltMon6"=789, "twVoltMon7"=790, "twVoltMon8"=791, "twVoltStat1"=792, "twVoltStat2"=793, "twVoltStat3"=794, "twVoltStat4"=795, "twVoltStat5"=796, "twVoltStat6"=797, "twVoltStat7"=798, "twVoltStat8"=799]
  in  "Wago Output Words 3":T1=832 items=["twHeatCtrl"=512, "twSteamCtrl"=513, "twCoolCtrl"=514, "twDehumCtrl"=515, "Output QX4 Bool"=516, "Output QX5 Bool"=517, "Output QX6 Bool"=518, "Output QX7 Bool"=519, "Output QX8 Bool"=520, "Output QX9 Bool"=521, "Output QX10"=522, "twRoomTemp"=840, "twRoomHum"=841, "twSuppTemp"=842, "twCoolTemp"=843, "twDehumTemp"=844, "twGlycolTemp"=845, "twHeatRate"=846, "twSteamRate"=847, "twCoolRate"=848, "twDehumRate"=849, "twStatus"=850, "twDoorEna"=851, "Rm1St1Dr1Stat"=816, "Rm1St2Dr1Stat"=817, "Rm1St3Dr1Stat"=818, "Rm1St4Dr1Stat"=819, "Rm1St5Dr1Stat"=820, "Rm1St6Dr1Stat"=821, "Rm1St7Dr1Stat"=822, "Rm1St8Dr1Stat"=823, "Rm1St1Dr2Stat"=824, "Rm1St2Dr2Stat"=825, "Rm1St3Dr2Stat"=826, "Rm1St4Dr2Stat"=827, "Rm1St5Dr2Stat"=828, "Rm1St6DrStat"=829, "Rm1St7Dr2Stat"=830, "Rm1St8Dr2Stat"=831, "Rm1St1Dr3Stat"=832, "Rm1St2Dr3Stat"=833, "Rm1St3Dr3Stat"=834, "Rm1St4Dr3Stat"=835, "Rm1St5Dr3Stat"=836, "Rm1St6Dr3Stat"=837, "Rm1St7Dr3Stat"=838, "Rm1St8Dr3Stat"=839, "twVoltMon1"=784, "twVoltMon2"=785, "twVoltMon3"=786, "twVoltMon4"=787, "twVoltMon5"=788, "twVoltMon6"=789, "twVoltMon7"=790, "twVoltMon8"=791, "twVoltStat1"=792, "twVoltStat2"=793, "twVoltStat3"=794, "twVoltStat4"=795, "twVoltStat5"=796, "twVoltStat6"=797, "twVoltStat7"=798, "twVoltStat8"=799]
  in  "Wago Output Words 2":T1=824 items=["twHeatCtrl"=512, "twSteamCtrl"=513, "twCoolCtrl"=514, "twDehumCtrl"=515, "Output QX4 Bool"=516, "Output QX5 Bool"=517, "Output QX6 Bool"=518, "Output QX7 Bool"=519, "Output QX8 Bool"=520, "Output QX9 Bool"=521, "Output QX10"=522, "twRoomTemp"=840, "twRoomHum"=841, "twSuppTemp"=842, "twCoolTemp"=843, "twDehumTemp"=844, "twGlycolTemp"=845, "twHeatRate"=846, "twSteamRate"=847, "twCoolRate"=848, "twDehumRate"=849, "twStatus"=850, "twDoorEna"=851, "Rm1St1Dr1Stat"=816, "Rm1St2Dr1Stat"=817, "Rm1St3Dr1Stat"=818, "Rm1St4Dr1Stat"=819, "Rm1St5Dr1Stat"=820, "Rm1St6Dr1Stat"=821, "Rm1St7Dr1Stat"=822, "Rm1St8Dr1Stat"=823, "Rm1St1Dr2Stat"=824, "Rm1St2Dr2Stat"=825, "Rm1St3Dr2Stat"=826, "Rm1St4Dr2Stat"=827, "Rm1St5Dr2Stat"=828, "Rm1St6DrStat"=829, "Rm1St7Dr2Stat"=830, "Rm1St8Dr2Stat"=831, "Rm1St1Dr3Stat"=832, "Rm1St2Dr3Stat"=833, "Rm1St3Dr3Stat"=834, "Rm1St4Dr3Stat"=835, "Rm1St5Dr3Stat"=836, "Rm1St6Dr3Stat"=837, "Rm1St7Dr3Stat"=838, "Rm1St8Dr3Stat"=839, "twVoltMon1"=784, "twVoltMon2"=785, "twVoltMon3"=786, "twVoltMon4"=787, "twVoltMon5"=788, "twVoltMon6"=789, "twVoltMon7"=790, "twVoltMon8"=791, "twVoltStat1"=792, "twVoltStat2"=793, "twVoltStat3"=794, "twVoltStat4"=795, "twVoltStat5"=796, "twVoltStat6"=797, "twVoltStat7"=798, "twVoltStat8"=799]
  in  "Wago Output Words":T1=816 items=["twHeatCtrl"=512, "twSteamCtrl"=513, "twCoolCtrl"=514, "twDehumCtrl"=515, "Output QX4 Bool"=516, "Output QX5 Bool"=517, "Output QX6 Bool"=518, "Output QX7 Bool"=519, "Output QX8 Bool"=520, "Output QX9 Bool"=521, "Output QX10"=522, "twRoomTemp"=840, "twRoomHum"=841, "twSuppTemp"=842, "twCoolTemp"=843, "twDehumTemp"=844, "twGlycolTemp"=845, "twHeatRate"=846, "twSteamRate"=847, "twCoolRate"=848, "twDehumRate"=849, "twStatus"=850, "twDoorEna"=851, "Rm1St1Dr1Stat"=816, "Rm1St2Dr1Stat"=817, "Rm1St3Dr1Stat"=818, "Rm1St4Dr1Stat"=819, "Rm1St5Dr1Stat"=820, "Rm1St6Dr1Stat"=821, "Rm1St7Dr1Stat"=822, "Rm1St8Dr1Stat"=823, "Rm1St1Dr2Stat"=824, "Rm1St2Dr2Stat"=825, "Rm1St3Dr2Stat"=826, "Rm1St4Dr2Stat"=827, "Rm1St5Dr2Stat"=828, "Rm1St6DrStat"=829, "Rm1St7Dr2Stat"=830, "Rm1St8Dr2Stat"=831, "Rm1St1Dr3Stat"=832, "Rm1St2Dr3Stat"=833, "Rm1St3Dr3Stat"=834, "Rm1St4Dr3Stat"=835, "Rm1St5Dr3Stat"=836, "Rm1St6Dr3Stat"=837, "Rm1St7Dr3Stat"=838, "Rm1St8Dr3Stat"=839, "twVoltMon1"=784, "twVoltMon2"=785, "twVoltMon3"=786, "twVoltMon4"=787, "twVoltMon5"=788, "twVoltMon6"=789, "twVoltMon7"=790, "twVoltMon8"=791, "twVoltStat1"=792, "twVoltStat2"=793, "twVoltStat3"=794, "twVoltStat4"=795, "twVoltStat5"=796, "twVoltStat6"=797, "twVoltStat7"=798, "twVoltStat8"=799]
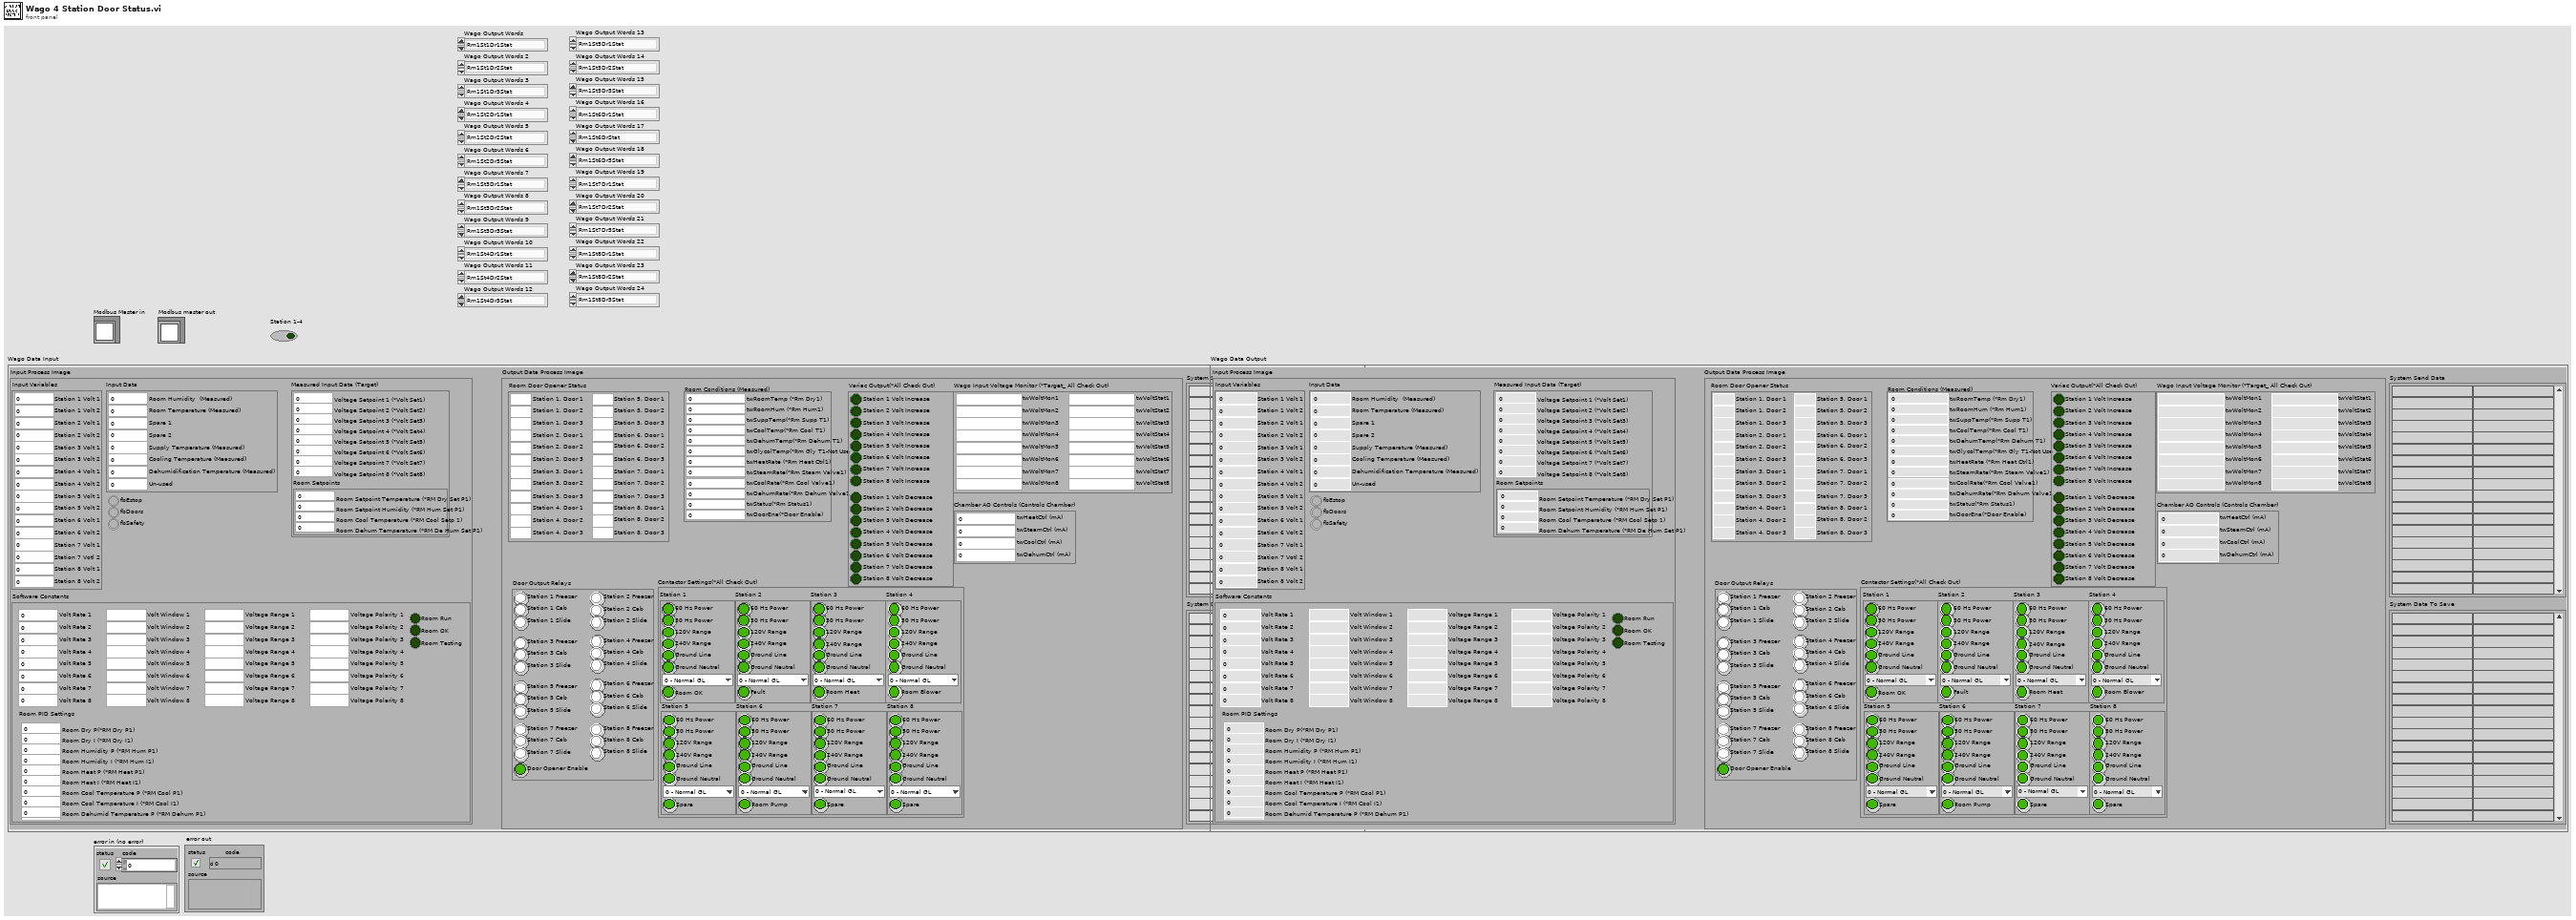
[diagram p1: front panel]
types:
  T1 = typedef "Wago Output Commands.ctl" = u16
  T2 = typedef "Wago Main Control.ctl" = cluster{"Output Data Process Image":T3, "Input Process Image":T8, "System Send Data":string[][], "System Data To Save":string[][]}
  T3 = typedef "Wago Output Data Process Image.ctl" = cluster{"Room Door Opener Status":cluster{"Station 1, Door 1":u16, "Station 1, Door 2":u16, "Station 1, Door 3":u16, "Station 2, Door 1":u16, "Station 2, Door 2":u16, "Station 2, Door 3":u16, "Station 3, Door 1":u16, "Station 3, Door 2":u16, "Station 3, Door 3":u16, "Station 4, Door 1":u16, "Station 4, Door 2":u16, "Station 4, Door 3":u16, "Station 5, Door 1":u16, "Station 5, Door 2":u16, "Station 5, Door 3":u16, "Station 6, Door 1":u16, "Station 6, Door 2":u16, "Station 6, Door 3":u16, "Station 7, Door 1":u16, "Station 7, Door 2":u16, "Station 7, Door 3":u16, "Station 8, Door 1":u16, "Station 8, Door 2":u16, "Station 8, Door 3":u16}, "Room Conditions (Measured)":T4, "Chamber AO Controls (Controls Chamber)":cluster{"twDehumCtrl (mA)":u16, "twCoolCtrl (mA)":u16, "twSteamCtrl (mA)":u16, "twHeatCtrl (mA)":u16}, "Variac Output(*All Check Out)":cluster{"Station 1 Volt Increase":bool, "Station 1 Volt Decrease":bool, "Station 2 Volt Increase":bool, "Station 2 Volt Decrease":bool, "Station 3 Volt Increase":bool, "Station 3 Volt Decrease":bool, "Station 4 Volt Increase":bool, "Station 4 Volt Decrease":bool, "Station 5 Volt Increase":bool, "Station 5 Volt Decrease":bool, "Station 6 Volt Increase":bool, "Station 6 Volt Decrease":bool, "Station 7 Volt Increase":bool, "Station 7 Volt Decrease":bool, "Station 8 Volt Increase":bool, "Station 8 Volt Decrease":bool}, "Door Output Relays":T5, "Wago Input Voltage Monitor (*Target_ All Check Out)":cluster{"twWoltMon1":dbl, "twWoltMon2":dbl, "twWoltMon3":dbl, "twWoltMon4":dbl, "twWoltMon5":dbl, "twWoltMon6":dbl, "twWoltMon7":dbl, "twWoltMon8":dbl, "twVoltStat1":u16, "twVoltStat2":u16, "twVoltStat3":u16, "twVoltStat4":u16, "twVoltStat5":u16, "twVoltStat6":u16, "twVoltStat7":u16, "twVoltStat8":u16}, "Contactor Settings(*All Check Out)":T6}
  T4 = typedef "Wago Room Condtions.ctl" = cluster{"twDoorEna(*Door Enable)":u16, "twStatus(*Rm Status1)":u16, "twRoomTemp (*Rm Dry1)":dbl, "twRoomHum (*Rm Hum1)":dbl, "twSuppTemp(*Rm Supp T1)":dbl, "twCoolTemp(*Rm Cool T1)":dbl, "twDehumTemp(*Rm Dehum T1)":dbl, "twGlycolTemp(*Rm Gly T1-Not Used)":dbl, "twDehumRate(*Rm Dehum Valve1)":dbl, "twCoolRate(*Rm Cool Valve1)":dbl, "twSteamRate(*Rm Steam Valve1)":dbl, "twHeatRate (*Rm Heat Ctrl1)":dbl}
  T5 = typedef "Wago Door Relays.ctl" = cluster{"Station 1 Freezer":bool, "Station 1 Cab":bool, "Station 1 Slide":bool, "Station 2 Freezer":bool, "Station 2 Cab":bool, "Station 2 Slide":bool, "Station 3 Freezer":bool, "Station 3 Cab":bool, "Station 3 Slide":bool, "Station 4 Freezer":bool, "Station 4 Cab":bool, "Station 4 Slide":bool, "Station 5 Freezer":bool, "Station 5 Cab":bool, "Station 5 Slide":bool, "Station 6 Freezer":bool, "Station 6 Cab":bool, "Station 6 Slide":bool, "Station 7 Freezer":bool, "Station 7 Cab":bool, "Station 7 Slide":bool, "Station 8 Freezer":bool, "Station 8 Cab":bool, "Station 8 Slide":bool, "Door Opener Enable":bool}
  T6 = typedef "Wago Contactor Settings.ctl" = cluster{"Station 1":cluster{"60 Hz Power":bool, "50 Hz Power":bool, "120V Range":bool, "240V Range":bool, "Ground Line":bool, "Ground Neutral":bool, "Room OK":bool, "Ground Leakage":T7}, "Station 2":cluster{"60 Hz Power":bool, "50 Hz Power":bool, "120V Range":bool, "240V Range":bool, "Ground Line":bool, "Ground Neutral":bool, "Fault":bool, "Ground Leakage":T7}, "Station 3":cluster{"60 Hz Power":bool, "50 Hz Power":bool, "120V Range":bool, "240V Range":bool, "Ground Line":bool, "Ground Neutral":bool, "Room Heat":bool, "Ground Leakage":T7}, "Station 4":cluster{"60 Hz Power":bool, "50 Hz Power":bool, "120V Range":bool, "240V Range":bool, "Ground Line":bool, "Ground Neutral":bool, "Room Blower":bool, "Ground Leakage":T7}, "Station 5":cluster{"60 Hz Power":bool, "50 Hz Power":bool, "120V Range":bool, "240V Range":bool, "Ground Line":bool, "Ground Neutral":bool, "Spare":bool, "Ground Leakage":T7}, "Station 6":cluster{"60 Hz Power":bool, "50 Hz Power":bool, "120V Range":bool, "240V Range":bool, "Ground Line":bool, "Ground Neutral":bool, "Room Pump":bool, "Ground Leakage":T7}, "Station 7":cluster{"60 Hz Power":bool, "50 Hz Power":bool, "120V Range":bool, "240V Range":bool, "Ground Line":bool, "Ground Neutral":bool, "Spare":bool, "Ground Leakage":T7}, "Station 8":cluster{"60 Hz Power":bool, "50 Hz Power":bool, "120V Range":bool, "240V Range":bool, "Ground Line":bool, "Ground Neutral":bool, "Spare":bool, "Ground Leakage":T7}}
  T7 = typedef "Wago Ground Leakage.ctl" = enum16{"0 - Normal GL", "1 - Measure GL"}
  T8 = typedef "Wago Input Process Image.ctl" = cluster{"fbEstop":bool, "fbDoors":bool, "fbSafety":bool, "Input Variables":cluster{"Station 1 Volt 1":dbl, "Station 1 Volt 2":dbl, "Station 2 Volt 1":dbl, "Station 2 Volt 2":dbl, "Station 3 Volt 1":dbl, "Station 3 Volt 2":dbl, "Station 4 Volt 1":dbl, "Station 4 Volt 2":dbl, "Station 5 Volt 1":dbl, "Station 5 Volt 2":dbl, "Station 6 Volt 1":dbl, "Station 6 Volt 2":dbl, "Station 7 Volt 1":dbl, "Station 7 Votl 2":dbl, "Station 8 Volt 1":dbl, "Station 8 Volt 2":dbl}, "Input Data":cluster{"Room Humidity  (Measured)":dbl, "Room Temperature (Measured)":dbl, "Spare 1":dbl, "Spare 2":dbl, "Supply Temperature (Measured)":dbl, "Cooling Temperature (Measured)":dbl, "Dehumidification Temperature (Measured)":dbl, "Un-used":dbl}, "Software Constants":cluster{"Volt Rate 1":u16, "Volt Rate 2":u16, "Volt Rate 3":u16, "Volt Rate 4":u16, "Volt Rate 5":u16, "Volt Rate 6":u16, "Volt Rate 7":u16, "Volt Rate 8":u16, "Volt Window 1":u16, "Volt Window 2":u16, "Volt Window 3":u16, "Volt Window 4":u16, "Volt Window 5":u16, "Volt Window 6":u16, "Volt Window 7":u16, "Volt Window 8":u16, "Voltage Range 1":u16, "Voltage Range 2":u16, "Voltage Range 3":u16, "Voltage Range 4":u16, "Voltage Range 5":u16, "Voltage Range 6":u16, "Voltage Range 7":u16, "Voltage Range 8":u16, "Voltage Polarity 1":u16, "Voltage Polarity 2":u16, "Voltage Polarity 3":u16, "Voltage Polarity 4":u16, "Voltage Polarity 5":u16, "Voltage Polarity 6":u16, "Voltage Polarity 7":u16, "Voltage Polarity 8":u16, "Room Run":bool, "Room OK":bool, "Room Testing":bool, "Room PID Settings":T9}, "Measured Input Data (Target)":T10}
  T9 = typedef "Wago Room PID Settings.ctl" = cluster{"Room Dry P(*RM Dry P1)":u16, "Room Dry I (*RM Dry I1)":u16, "Room Humidity P (*RM Hum P1)":u16, "Room Humidity I (*RM Hum I1)":u16, "Room Heat P (*RM Heat P1)":u16, "Room Heat I (*RM Heat I1)":u16, "Room Cool Temperature P (*RM Cool P1)":u16, "Room Cool Temperature I (*RM Cool I1)":u16, "Room Dehumid Temperature P (*RM Dehum P1)":u16, "Room Dehumid Temperature I (*RM Dehum I1)":u16}
  T10 = typedef "Wago Measured Input Data.ctl" = cluster{"Voltage Setpoint 1 (*Volt Set1)":dbl, "Voltage Setpoint 2 (*Volt Set2)":dbl, "Voltage Setpoint 3 (*Volt Set3)":dbl, "Voltage Setpoint 4 (*Volt Set4)":dbl, "Voltage Setpoint 5 (*Volt Set5)":dbl, "Voltage Setpoint 6 (*Volt Set6)":dbl, "Voltage Setpoint 7 (*Volt Set7)":dbl, "Voltage Setpoint 8 (*Volt Set8)":dbl, "Room Setpoints":T11}
  T11 = typedef "Wago Room Setpoint Targets.ctl" = cluster{"Room Setpoint Temperature (*RM Dry Set P1)":dbl, "Room Setpoint Humidity (*RM Hum Set P1)":dbl, "Room Cool Temperature (*RM Cool Setp 1)":dbl, "Room Dehum Temperature (*RM De Hum Set P1)":dbl}
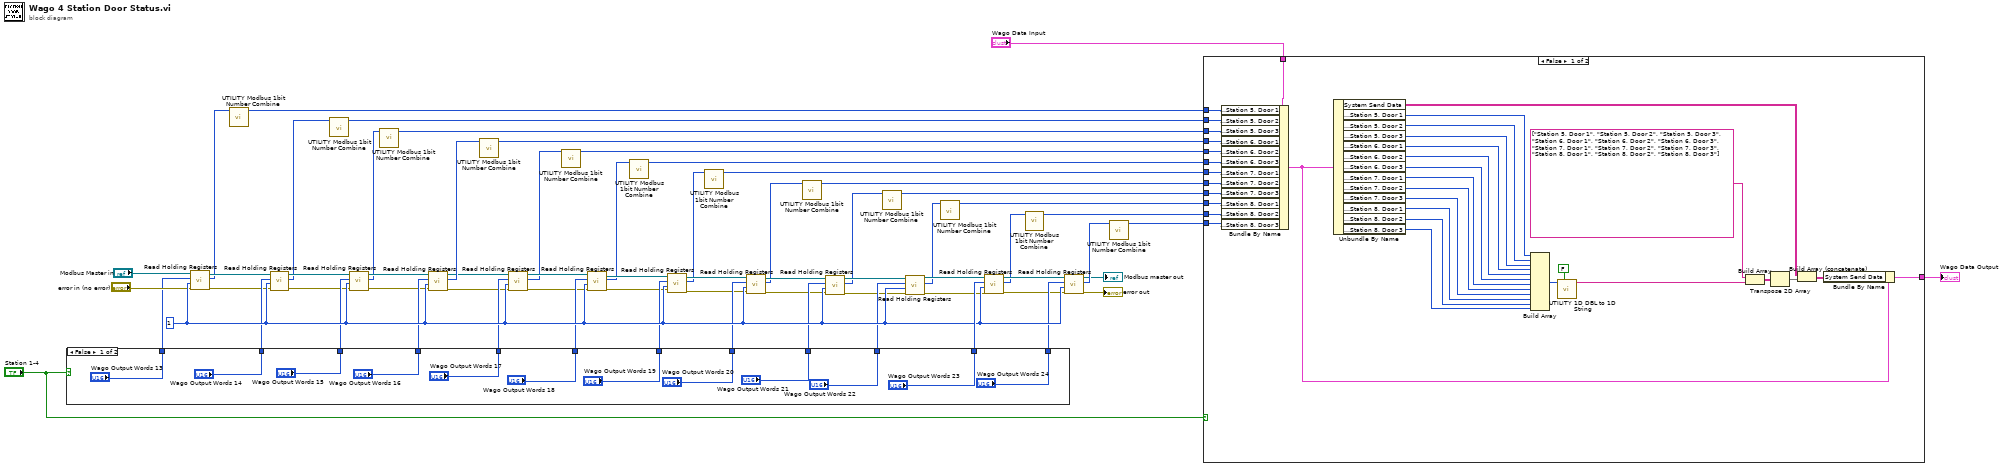
[diagram p0: block diagram]
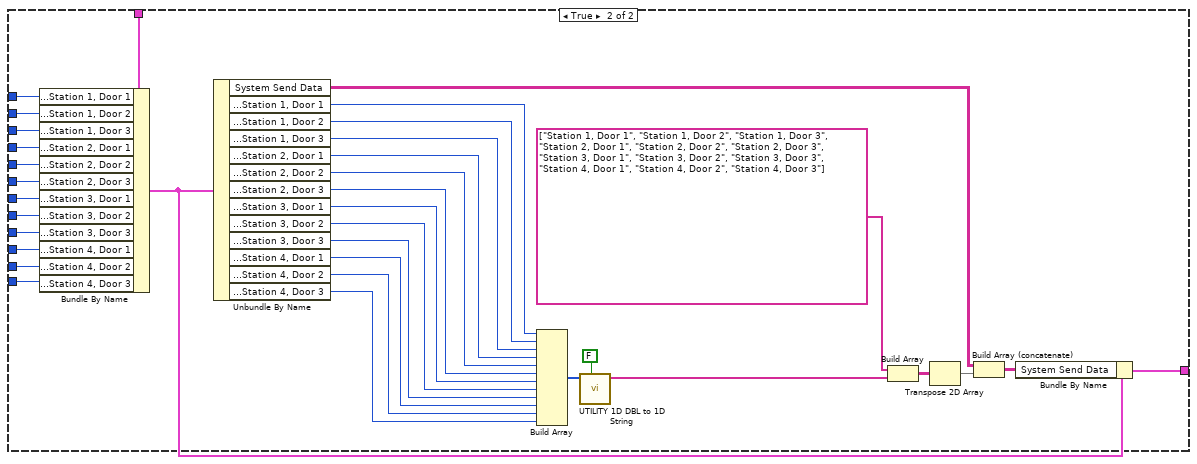
[diagram p2: hidden frame]
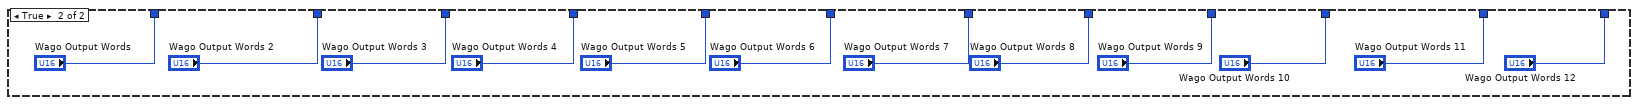
[diagram p3: hidden frame]
diagram:
  w52 = u16 1 ("Quantity")
  n1 = case shown="False" "Station 1-4" {
    tunnel: ["Wago Output Words 23" "Wago Output Words 11"] -> w66
    tunnel: ["Wago Output Words 24" "Wago Output Words 12"] -> w51
    tunnel: ["Wago Output Words 22" "Wago Output Words 10"] -> w44
    tunnel: ["Wago Output Words 21" "Wago Output Words 9"] -> w40
    tunnel: ["Wago Output Words 20" "Wago Output Words 8"] -> w36
    tunnel: ["Wago Output Words 19" "Wago Output Words 7"] -> w32
    tunnel: ["Wago Output Words 18" "Wago Output Words 6"] -> w28
    tunnel: ["Wago Output Words 17" "Wago Output Words 5"] -> w24
    tunnel: ["Wago Output Words 16" "Wago Output Words 4"] -> w20
    tunnel: ["Wago Output Words 15" "Wago Output Words 3"] -> w16
    tunnel: ["Wago Output Words 14" "Wago Output Words 2"] -> w13
    tunnel: ["Wago Output Words 13" "Wago Output Words"] -> w7
    frame False {
    }
    frame True {
    }
  }
  n2 = call-dynamic "Read Holding Registers.vi"("error in"="error in (no error)", "number of inputs"=w52, "starting address"=w7, "Modbus master in"="Modbus Master in") -> ("error out"=w10:errorcluster, "register values"=w8:u16[], "Modbus master out"=w11:refnum<class "Modbus Master.lvclass">)  [unwired: 5 in]
  n3 = call "UTILITY Modbus 1bit Number Combine.vi"("register values"=w8) -> ("Data"=w54:u16)  [unwired: 10 in]
  n4 = call-dynamic "Read Holding Registers.vi"("error in"=w10, "number of inputs"=w52, "starting address"=w13, "Modbus master in"=w11) -> ("error out"=w14:errorcluster, "register values"=w12:u16[], "Modbus master out"=w15:refnum<class "Modbus Master.lvclass">)  [unwired: 5 in]
  n5 = call "UTILITY Modbus 1bit Number Combine.vi"("register values"=w12) -> ("Data"=w55:u16)  [unwired: 10 in]
  n6 = call-dynamic "Read Holding Registers.vi"("error in"=w14, "number of inputs"=w52, "starting address"=w16, "Modbus master in"=w15) -> ("error out"=w18:errorcluster, "register values"=w17:u16[], "Modbus master out"=w19:refnum<class "Modbus Master.lvclass">)  [unwired: 5 in]
  n7 = call "UTILITY Modbus 1bit Number Combine.vi"("register values"=w17) -> ("Data"=w56:u16)  [unwired: 10 in]
  n8 = call-dynamic "Read Holding Registers.vi"("error in"=w18, "number of inputs"=w52, "starting address"=w20, "Modbus master in"=w19) -> ("error out"=w21:errorcluster, "register values"=w23:u16[], "Modbus master out"=w22:refnum<class "Modbus Master.lvclass">)  [unwired: 5 in]
  n9 = call "UTILITY Modbus 1bit Number Combine.vi"("register values"=w23) -> ("Data"=w57:u16)  [unwired: 10 in]
  n10 = call-dynamic "Read Holding Registers.vi"("error in"=w21, "number of inputs"=w52, "starting address"=w24, "Modbus master in"=w22) -> ("error out"=w27:errorcluster, "register values"=w25:u16[], "Modbus master out"=w26:refnum<class "Modbus Master.lvclass">)  [unwired: 5 in]
  n11 = call "UTILITY Modbus 1bit Number Combine.vi"("register values"=w25) -> ("Data"=w58:u16)  [unwired: 10 in]
  n12 = call-dynamic "Read Holding Registers.vi"("error in"=w27, "number of inputs"=w52, "starting address"=w28, "Modbus master in"=w26) -> ("error out"=w30:errorcluster, "register values"=w29:u16[], "Modbus master out"=w31:refnum<class "Modbus Master.lvclass">)  [unwired: 5 in]
  n13 = call "UTILITY Modbus 1bit Number Combine.vi"("register values"=w29) -> ("Data"=w59:u16)  [unwired: 10 in]
  n14 = call-dynamic "Read Holding Registers.vi"("error in"=w30, "number of inputs"=w52, "starting address"=w32, "Modbus master in"=w31) -> ("error out"=w34:errorcluster, "register values"=w33:u16[], "Modbus master out"=w35:refnum<class "Modbus Master.lvclass">)  [unwired: 5 in]
  n15 = call "UTILITY Modbus 1bit Number Combine.vi"("register values"=w33) -> ("Data"=w60:u16)  [unwired: 10 in]
  n16 = call-dynamic "Read Holding Registers.vi"("error in"=w34, "number of inputs"=w52, "starting address"=w36, "Modbus master in"=w35) -> ("error out"=w38:errorcluster, "register values"=w37:u16[], "Modbus master out"=w39:refnum<class "Modbus Master.lvclass">)  [unwired: 5 in]
  n17 = call "UTILITY Modbus 1bit Number Combine.vi"("register values"=w37) -> ("Data"=w61:u16)  [unwired: 10 in]
  n18 = call-dynamic "Read Holding Registers.vi"("error in"=w38, "number of inputs"=w52, "starting address"=w40, "Modbus master in"=w39) -> ("error out"=w43:errorcluster, "register values"=w41:u16[], "Modbus master out"=w42:refnum<class "Modbus Master.lvclass">)  [unwired: 5 in]
  n19 = call "UTILITY Modbus 1bit Number Combine.vi"("register values"=w41) -> ("Data"=w62:u16)  [unwired: 10 in]
  n20 = call-dynamic "Read Holding Registers.vi"("error in"=w43, "number of inputs"=w52, "starting address"=w44, "Modbus master in"=w42) -> ("error out"=w46:errorcluster, "register values"=w45:u16[], "Modbus master out"=w47:refnum<class "Modbus Master.lvclass">)  [unwired: 5 in]
  n21 = call "UTILITY Modbus 1bit Number Combine.vi"("register values"=w45) -> ("Data"=w63:u16)  [unwired: 10 in]
  n22 = call-dynamic "Read Holding Registers.vi"("error in"=w46, "number of inputs"=w52, "starting address"=w66, "Modbus master in"=w47) -> ("error out"=w49:errorcluster, "register values"=w48:u16[], "Modbus master out"=w50:refnum<class "Modbus Master.lvclass">)  [unwired: 5 in]
  n23 = call "UTILITY Modbus 1bit Number Combine.vi"("register values"=w48) -> ("Data"=w64:u16)  [unwired: 10 in]
  n24 = call-dynamic "Read Holding Registers.vi"("error in"=w49, "number of inputs"=w52, "starting address"=w51, "Modbus master in"=w50) -> ("error out"=→"error out":errorcluster, "register values"=w53:u16[], "Modbus master out"=→"Modbus master out":refnum<class "Modbus Master.lvclass">)  [unwired: 5 in]
  n25 = call "UTILITY Modbus 1bit Number Combine.vi"("register values"=w53) -> ("Data"=w65:u16)  [unwired: 10 in]
  n26 = case shown="False" "Station 1-4" {
    tunnel: w65 -> [w113 w160]
    tunnel: w64 -> [w114 w159]
    tunnel: w63 -> [w115 w158]
    tunnel: w62 -> [w116 w157]
    tunnel: w61 -> [w117 w156]
    tunnel: w60 -> [w118 w155]
    tunnel: w59 -> [w119 w154]
    tunnel: w58 -> [w120 w153]
    tunnel: w57 -> [w121 w152]
    tunnel: w56 -> [w122 w151]
    tunnel: w55 -> [w123 w150]
    tunnel: w54 -> [w124 w149]
    tunnel: [w103 w137] -> w1
    tunnel: "Wago Data Input" -> [w125 w148]
    frame False {
      n27 = Bundle By Name(cluster=w125, "Output Data Process Image.Room Door Opener Status.Station 5, Door 1"=w124, "Output Data Process Image.Room Door Opener Status.Station 5, Door 2"=w123, "Output Data Process Image.Room Door Opener Status.Station 5, Door 3"=w122, "Output Data Process Image.Room Door Opener Status.Station 6, Door 1"=w121, "Output Data Process Image.Room Door Opener Status.Station 6, Door 2"=w120, "Output Data Process Image.Room Door Opener Status.Station 6, Door 3"=w119, "Output Data Process Image.Room Door Opener Status.Station 7, Door 1"=w118, "Output Data Process Image.Room Door Opener Status.Station 7, Door 2"=w117, "Output Data Process Image.Room Door Opener Status.Station 7, Door 3"=w116, "Output Data Process Image.Room Door Opener Status.Station 8, Door 1"=w115, "Output Data Process Image.Room Door Opener Status.Station 8, Door 2"=w114, "Output Data Process Image.Room Door Opener Status.Station 8, Door 3"=w113) -> (w102:T2)
      n28 = Unbundle By Name(w102) -> ("System Send Data"=w110:string[][], "Output Data Process Image.Room Door Opener Status.Station 5, Door 1"=w105:u16, "Output Data Process Image.Room Door Opener Status.Station 5, Door 2"=w101:u16, "Output Data Process Image.Room Door Opener Status.Station 5, Door 3"=w100:u16, "Output Data Process Image.Room Door Opener Status.Station 6, Door 1"=w99:u16, "Output Data Process Image.Room Door Opener Status.Station 6, Door 2"=w98:u16, "Output Data Process Image.Room Door Opener Status.Station 6, Door 3"=w97:u16, "Output Data Process Image.Room Door Opener Status.Station 7, Door 1"=w96:u16, "Output Data Process Image.Room Door Opener Status.Station 7, Door 2"=w95:u16, "Output Data Process Image.Room Door Opener Status.Station 7, Door 3"=w94:u16, "Output Data Process Image.Room Door Opener Status.Station 8, Door 1"=w93:u16, "Output Data Process Image.Room Door Opener Status.Station 8, Door 2"=w92:u16, "Output Data Process Image.Room Door Opener Status.Station 8, Door 3"=w91:u16)
      n29 = Build Array(w105, w101, w100, w99, w98, w97, w96, w95, w94, w93, w92, w91) -> (w106:u16[])
      n30 = call "UTILITY 1D DBL to 1D String.vi"("DBL?"=FALSE, "1D DBL"=w106) -> ("1D String"=w108:string[])  [unwired: 9 in]
      n31 = Build Array(string[] ["Station 5, Door 1", "Station 5, Door 2", "Station 5, Door 3", "Station 6, Door 1", "Station 6, Door 2", "Station 6, Door 3", "Station 7, Door 1", "Station 7, Door 2", "Station 7, Door 3", "Station 8, Door 1", "Station 8, Door 2", "Station 8, Door 3"], w108) -> (w109:string[][])
      n32 = Transpose 2D Array(2D array=w109) -> (transposed array=w111:string[][])
      n33 = Build Array (concatenate)(w110, w111) -> (w112:string[][])
      n34 = Bundle By Name(cluster=w102, "System Send Data"=w112) -> (w103:T2)
    }
    frame True {
      n35 = Bundle By Name(cluster=w148, "Output Data Process Image.Room Door Opener Status.Station 1, Door 1"=w149, "Output Data Process Image.Room Door Opener Status.Station 1, Door 2"=w150, "Output Data Process Image.Room Door Opener Status.Station 1, Door 3"=w151, "Output Data Process Image.Room Door Opener Status.Station 2, Door 1"=w152, "Output Data Process Image.Room Door Opener Status.Station 2, Door 2"=w153, "Output Data Process Image.Room Door Opener Status.Station 2, Door 3"=w154, "Output Data Process Image.Room Door Opener Status.Station 3, Door 1"=w155, "Output Data Process Image.Room Door Opener Status.Station 3, Door 2"=w156, "Output Data Process Image.Room Door Opener Status.Station 3, Door 3"=w157, "Output Data Process Image.Room Door Opener Status.Station 4, Door 1"=w158, "Output Data Process Image.Room Door Opener Status.Station 4, Door 2"=w159, "Output Data Process Image.Room Door Opener Status.Station 4, Door 3"=w160) -> (w138:T2)
      n36 = Unbundle By Name(w138) -> ("System Send Data"=w145:string[][], "Output Data Process Image.Room Door Opener Status.Station 1, Door 1"=w140:u16, "Output Data Process Image.Room Door Opener Status.Station 1, Door 2"=w136:u16, "Output Data Process Image.Room Door Opener Status.Station 1, Door 3"=w135:u16, "Output Data Process Image.Room Door Opener Status.Station 2, Door 1"=w134:u16, "Output Data Process Image.Room Door Opener Status.Station 2, Door 2"=w133:u16, "Output Data Process Image.Room Door Opener Status.Station 2, Door 3"=w132:u16, "Output Data Process Image.Room Door Opener Status.Station 3, Door 1"=w131:u16, "Output Data Process Image.Room Door Opener Status.Station 3, Door 2"=w130:u16, "Output Data Process Image.Room Door Opener Status.Station 3, Door 3"=w129:u16, "Output Data Process Image.Room Door Opener Status.Station 4, Door 1"=w128:u16, "Output Data Process Image.Room Door Opener Status.Station 4, Door 2"=w127:u16, "Output Data Process Image.Room Door Opener Status.Station 4, Door 3"=w126:u16)
      n37 = Build Array(w140, w136, w135, w134, w133, w132, w131, w130, w129, w128, w127, w126) -> (w141:u16[])
      n38 = call "UTILITY 1D DBL to 1D String.vi"("DBL?"=FALSE, "1D DBL"=w141) -> ("1D String"=w143:string[])  [unwired: 9 in]
      n39 = Build Array(string[] ["Station 1, Door 1", "Station 1, Door 2", "Station 1, Door 3", "Station 2, Door 1", "Station 2, Door 2", "Station 2, Door 3", "Station 3, Door 1", "Station 3, Door 2", "Station 3, Door 3", "Station 4, Door 1", "Station 4, Door 2", "Station 4, Door 3"], w143) -> (w144:string[][])
      n40 = Transpose 2D Array(2D array=w144) -> (transposed array=w146:string[][])
      n41 = Build Array (concatenate)(w145, w146) -> (w147:string[][])
      n42 = Bundle By Name(cluster=w138, "System Send Data"=w147) -> (w137:T2)
    }
  }
  "Wago Data Output" <- w1
